vi "Writer.vi"(9 "output cluster":T1, 10 "FileName":string="Blue2.csv", 11 "FilePath":path=path "C:/Program Files (x86)/FRC Dashboard") -> ()   [LabVIEW 2013]
panel:
  in  "Color Components":T2={"Hue"={110.0, 142.0}, "Sat"={138.0, 255.0}, "Val"={139.0, 198.0}} {"Val" scale=0.0..255.0; "Sat" scale=0.0..255.0; "Hue" scale=0.0..255.0 scale format="%#_3g"}
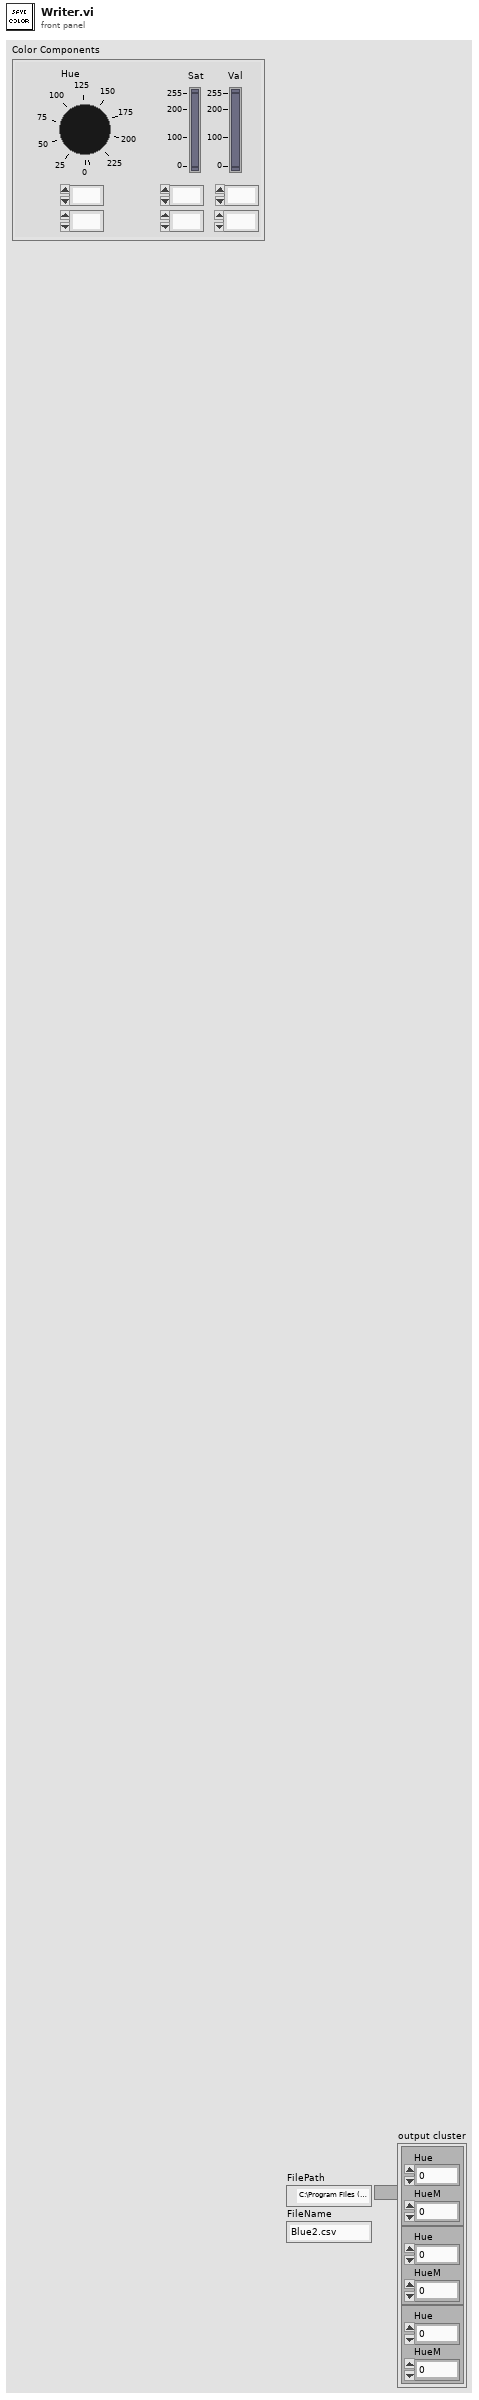
[diagram p1: front panel]
types:
  T1 = cluster{cluster{"Hue":i32, "HueM":i32}, cluster{"Hue":i32, "HueM":i32}, cluster{"Hue":i32, "HueM":i32}}
  T2 = cluster{"Hue":cluster{dbl, dbl}, "Sat":cluster{dbl, dbl}, "Val":cluster{dbl, dbl}}
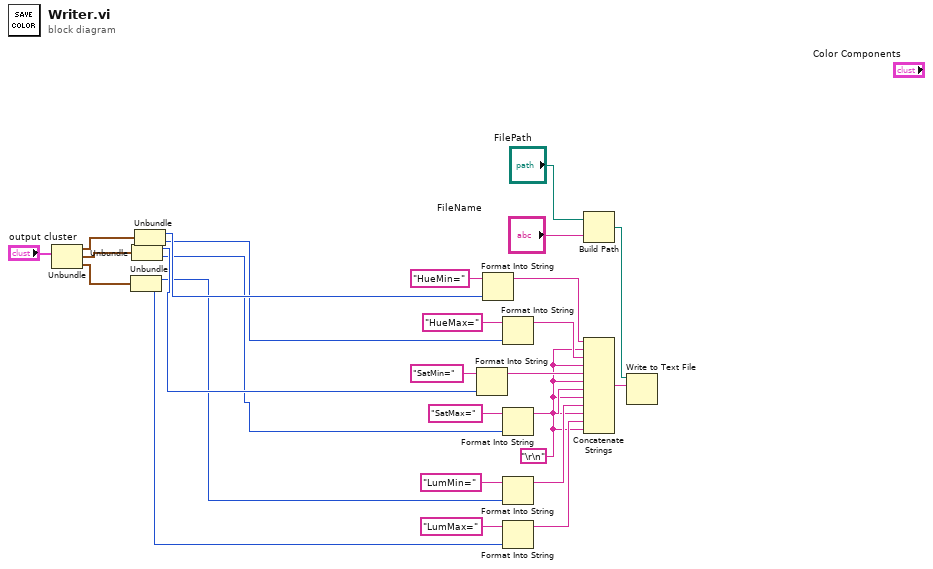
[diagram p0: block diagram]
diagram:
  w13 = "\r\n"
  n1 = Unbundle("output cluster") -> (w9:cluster{"Hue":i32, "HueM":i32}, w8:cluster{"Hue":i32, "HueM":i32}, w7:cluster{"Hue":i32, "HueM":i32})
  n2 = Unbundle(w7) -> ("Hue"=w2:i32, "HueM"=w1:i32)
  n3 = Unbundle(w8) -> ("Hue"=w4:i32, "HueM"=w3:i32)
  n4 = Unbundle(w9) -> ("Hue"=w6:i32, "HueM"=w5:i32)
  n5 = Format Into String(initial string="SatMin=", w4) -> (resulting string=w16:string)  [unwired: 2 in, 1 out]
  n6 = Format Into String(initial string="HueMin=", w6) -> (resulting string=w26:string)  [unwired: 2 in, 1 out]
  n7 = Format Into String(initial string="HueMax=", w5) -> (resulting string=w24:string)  [unwired: 2 in, 1 out]
  n8 = Format Into String(initial string="SatMax=", w3) -> (resulting string=w21:string)  [unwired: 2 in, 1 out]
  n9 = Format Into String(initial string="LumMin=", w2) -> (resulting string=w15:string)  [unwired: 2 in, 1 out]
  n10 = Format Into String(initial string="LumMax=", w1) -> (resulting string=w14:string)  [unwired: 2 in, 1 out]
  n11 = Build Path(base path="FilePath", name or relative path="FileName") -> (appended path=w11:path)
  n12 = Concatenate Strings(w26, w13, w24, w13, w16, w13, w21, w13, w15, w13, w14, w13) -> (w12:string)
  n13 = Write to Text File(file (use dialog)=w11, text=w12) -> ()  [unwired: 2 in, 3 out]
